vi "AccelerometerBK.vi"() -> ()   [LabVIEW 2016]
uses:
  AccelerometerSample.ctl
  Telemetry/TelemetryDataTypes.ctl
  Telemetry/TelemetryUpdateModes.ctl
  Telemetry/TelemetryFields.ctl
  <vilib>/rvi/eio/common/nirviEmuTemplateMethod_errors.vi
  <vilib>/rvi/Emulation/niFpgaGetClockAttributes.vi
  <vilib>/rvi/Emulation/niFpgaSctlEmulationGetInTimedLoop.vi
  <vilib>/rvi/Emulation/niFpgaEmulationReportErrorSimple.vi
  <vilib>/rvi/Emulation/niFpgaEmulationIsFPGAContextNoSignature.vi
  <vilib>/rvi/errors/niFpgaSetErrorForExecOnDevCompSimple.vi
  <vilib>/rvi/eio/common/nirviEmuReportErrorAndStop.vi
  <vilib>/rvi/DataTransferAndStorage/Container/Common/niFpgaContainerGetUniqueNameForEmu.vi
  <vilib>/rvi/FIFO/Fifo_Resource/nirvififoEmulationSetSize.vi
  <vilib>/rvi/FIFO/Fifo_Resource/nirviFifoEmulationQueueMgr.vi
  <instcachedir>/0/nirviFifoEmulationQueueMgr_E5CAEC123FF24DC58D834DCA3CDAA9B5.lvgen/nirviFifoEmulationQueueMgr_E5CAEC123FF24DC58D834DCA3CDAA9B5_004.vi
  <vilib>/Utility/error.llb/Clear Errors.vi
  <vilib>/rvi/FIFO/Fifo_Resource/nirvififoEmulationCreateLock.vi
  <vilib>/rvi/Emulation/niFpgaProcessEmulError.vi
  <vilib>/rvi/FIFO/Fifo_Resource/nirvififoEmulationObtainLock.vi
  <vilib>/rvi/FIFO/Fifo_Resource/nirvififoEmulationReleaseLock.vi
  <vilib>/rvi/occurrence/nirviWaitOnOccurrenceBase.vi
  <vilib>/rvi/errors/nirviReportUnexpectedCaseInternalError.vi
  <vilib>/rvi/errors/nirviReportUnexpectedCaseInternalError (U32).vi
  <instcachedir>/0/nirviFifoEmulationQueueMgr_E5CAEC123FF24DC58D834DCA3CDAA9B5.lvgen/nirviFifoEmulationQueueMgr_E5CAEC123FF24DC58D834DCA3CDAA9B5_026.vi
  <vilib>/rvi/FIFO/Fifo_Resource/nirvififoEmulationDetermineInputValidOut.vi
  <vilib>/rvi/Emulation/niFpgaCriticalErrorInLSC.vi
  <userlib>/_NI FLP Library/FPGA/outsideSCTL/FlpLib Multiply Shared Instance 0.vi
  <userlib>/_NI FLP Library/FPGA/outsideSCTL/FlpLib Add Shared Instance 0.vi
  <userlib>/_NI FLP Library/FPGA/outsideSCTL/FlpLib Subtract Shared Instance 0.vi
  <userlib>/_NI FLP Library/FPGA/outsideSCTL/FlpLib Divide Shared Instance 0.vi
  <instcachedir>/0/nirviFifoEmulationQueueMgr_E5CAEC123FF24DC58D834DCA3CDAA9B5.lvgen/nirviFifoEmulationQueueMgr_E5CAEC123FF24DC58D834DCA3CDAA9B5_024.vi
  <instcachedir>/0/nirviFifoEmulationQueueMgr_E5CAEC123FF24DC58D834DCA3CDAA9B5.lvgen/nirviFifoEmulationQueueMgr_E5CAEC123FF24DC58D834DCA3CDAA9B5_025.vi
  <vilib>/eio/EIONode/EIONode.xnode
  <vilib>/rvi/DataTransferAndStorage/Container/XNode/niFpgaContainer.xnode
  <vilib>/rvi/FIFO/Fifo_Resource/nirvififoEmulationRead.vi
  <vilib>/rvi/FIFO/Fifo_Resource/nirvififoEmulationWrite.vi
panel:
  out "Memory":T1
  out "Data":T1
  out "Sample":T2
  out "Acceleration":T1
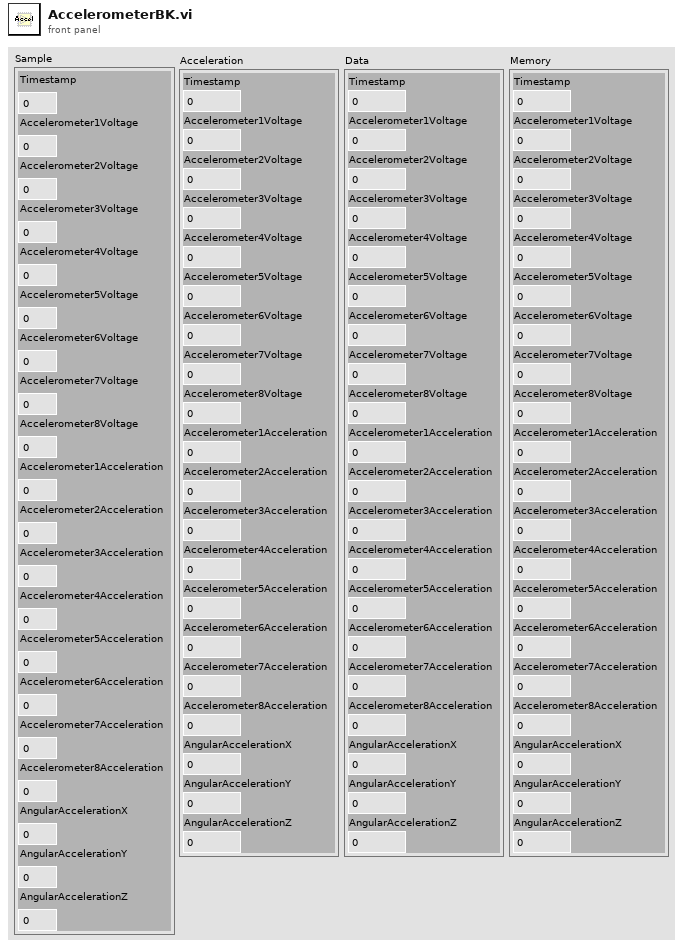
[diagram p1: front panel]
types:
  T1 = cluster{"Timestamp":u64, "Accelerometer1Voltage":sgl, "Accelerometer2Voltage":sgl, "Accelerometer3Voltage":sgl, "Accelerometer4Voltage":sgl, "Accelerometer5Voltage":sgl, "Accelerometer6Voltage":sgl, "Accelerometer7Voltage":sgl, "Accelerometer8Voltage":sgl, "Accelerometer1Acceleration":sgl, "Accelerometer2Acceleration":sgl, "Accelerometer3Acceleration":sgl, "Accelerometer4Acceleration":sgl, "Accelerometer5Acceleration":sgl, "Accelerometer6Acceleration":sgl, "Accelerometer7Acceleration":sgl, "Accelerometer8Acceleration":sgl, "AngularAccelerationX":sgl, "AngularAccelerationY":sgl, "AngularAccelerationZ":sgl}
  T2 = typedef "AccelerometerSample.ctl" = cluster{"Timestamp":u64, "Accelerometer1Voltage":sgl, "Accelerometer2Voltage":sgl, "Accelerometer3Voltage":sgl, "Accelerometer4Voltage":sgl, "Accelerometer5Voltage":sgl, "Accelerometer6Voltage":sgl, "Accelerometer7Voltage":sgl, "Accelerometer8Voltage":sgl, "Accelerometer1Acceleration":sgl, "Accelerometer2Acceleration":sgl, "Accelerometer3Acceleration":sgl, "Accelerometer4Acceleration":sgl, "Accelerometer5Acceleration":sgl, "Accelerometer6Acceleration":sgl, "Accelerometer7Acceleration":sgl, "Accelerometer8Acceleration":sgl, "AngularAccelerationX":sgl, "AngularAccelerationY":sgl, "AngularAccelerationZ":sgl}
  T3 = typedef "TelemetryFields.ctl" = enum16{"InclinometerErrorCode", "InclinometerTxBytes", "InclinometerRxBytes", "InclinometerTxFrames", "InclinometerRxFrames", "InclinometerTimestamp", "InclinometerAngle", "DisplacementErrorCode", "DisplacementTxBytes", "DisplacementRxBytes", "DisplacementTxFrames", "DisplacementRxFrames", "DisplacementTimestamp", "Displacement1", "Displacement2", "Displacement3", "Displacement4", "Displacement5", "Displacement6", "Displacement7", "Displacement8", "AccelerometerSampleCount", "AccelerometerTimestamp", "AccelerometerRaw1", "AccelerometerRaw2", "AccelerometerRaw3", "AccelerometerRaw4", "AccelerometerRaw5", "AccelerometerRaw6", "AccelerometerRaw7", "AccelerometerRaw8", "AccelerometerEng1", "AccelerometerEng2", "AccelerometerEng3", "AccelerometerEng4", "AccelerometerEng5", "AccelerometerEng6", "AccelerometerEng7", "AccelerometerEng8", "AngularAccelerationX", "AngularAccelerationY", "AngularAccelerationZ"}
  T4 = typedef "TelemetryUpdateModes.ctl" = enum8{"=", "+", "-", "|"}
  T5 = typedef "TelemetryDataTypes.ctl" = enum8{"U8", "U16", "U32", "U64", "I8", "I16", "I32", "I64", "SGL"}
  T6 = typedef "TelemetryUpdateData.ctl" = cluster{"DataType":T5, "Mode":T4, "Field":T3, "Data":u64}
  T7 = typedef "TelemetryUpdateDataSGL.ctl" = cluster{"Mode":T4, "Field":T3, "Data":sgl}
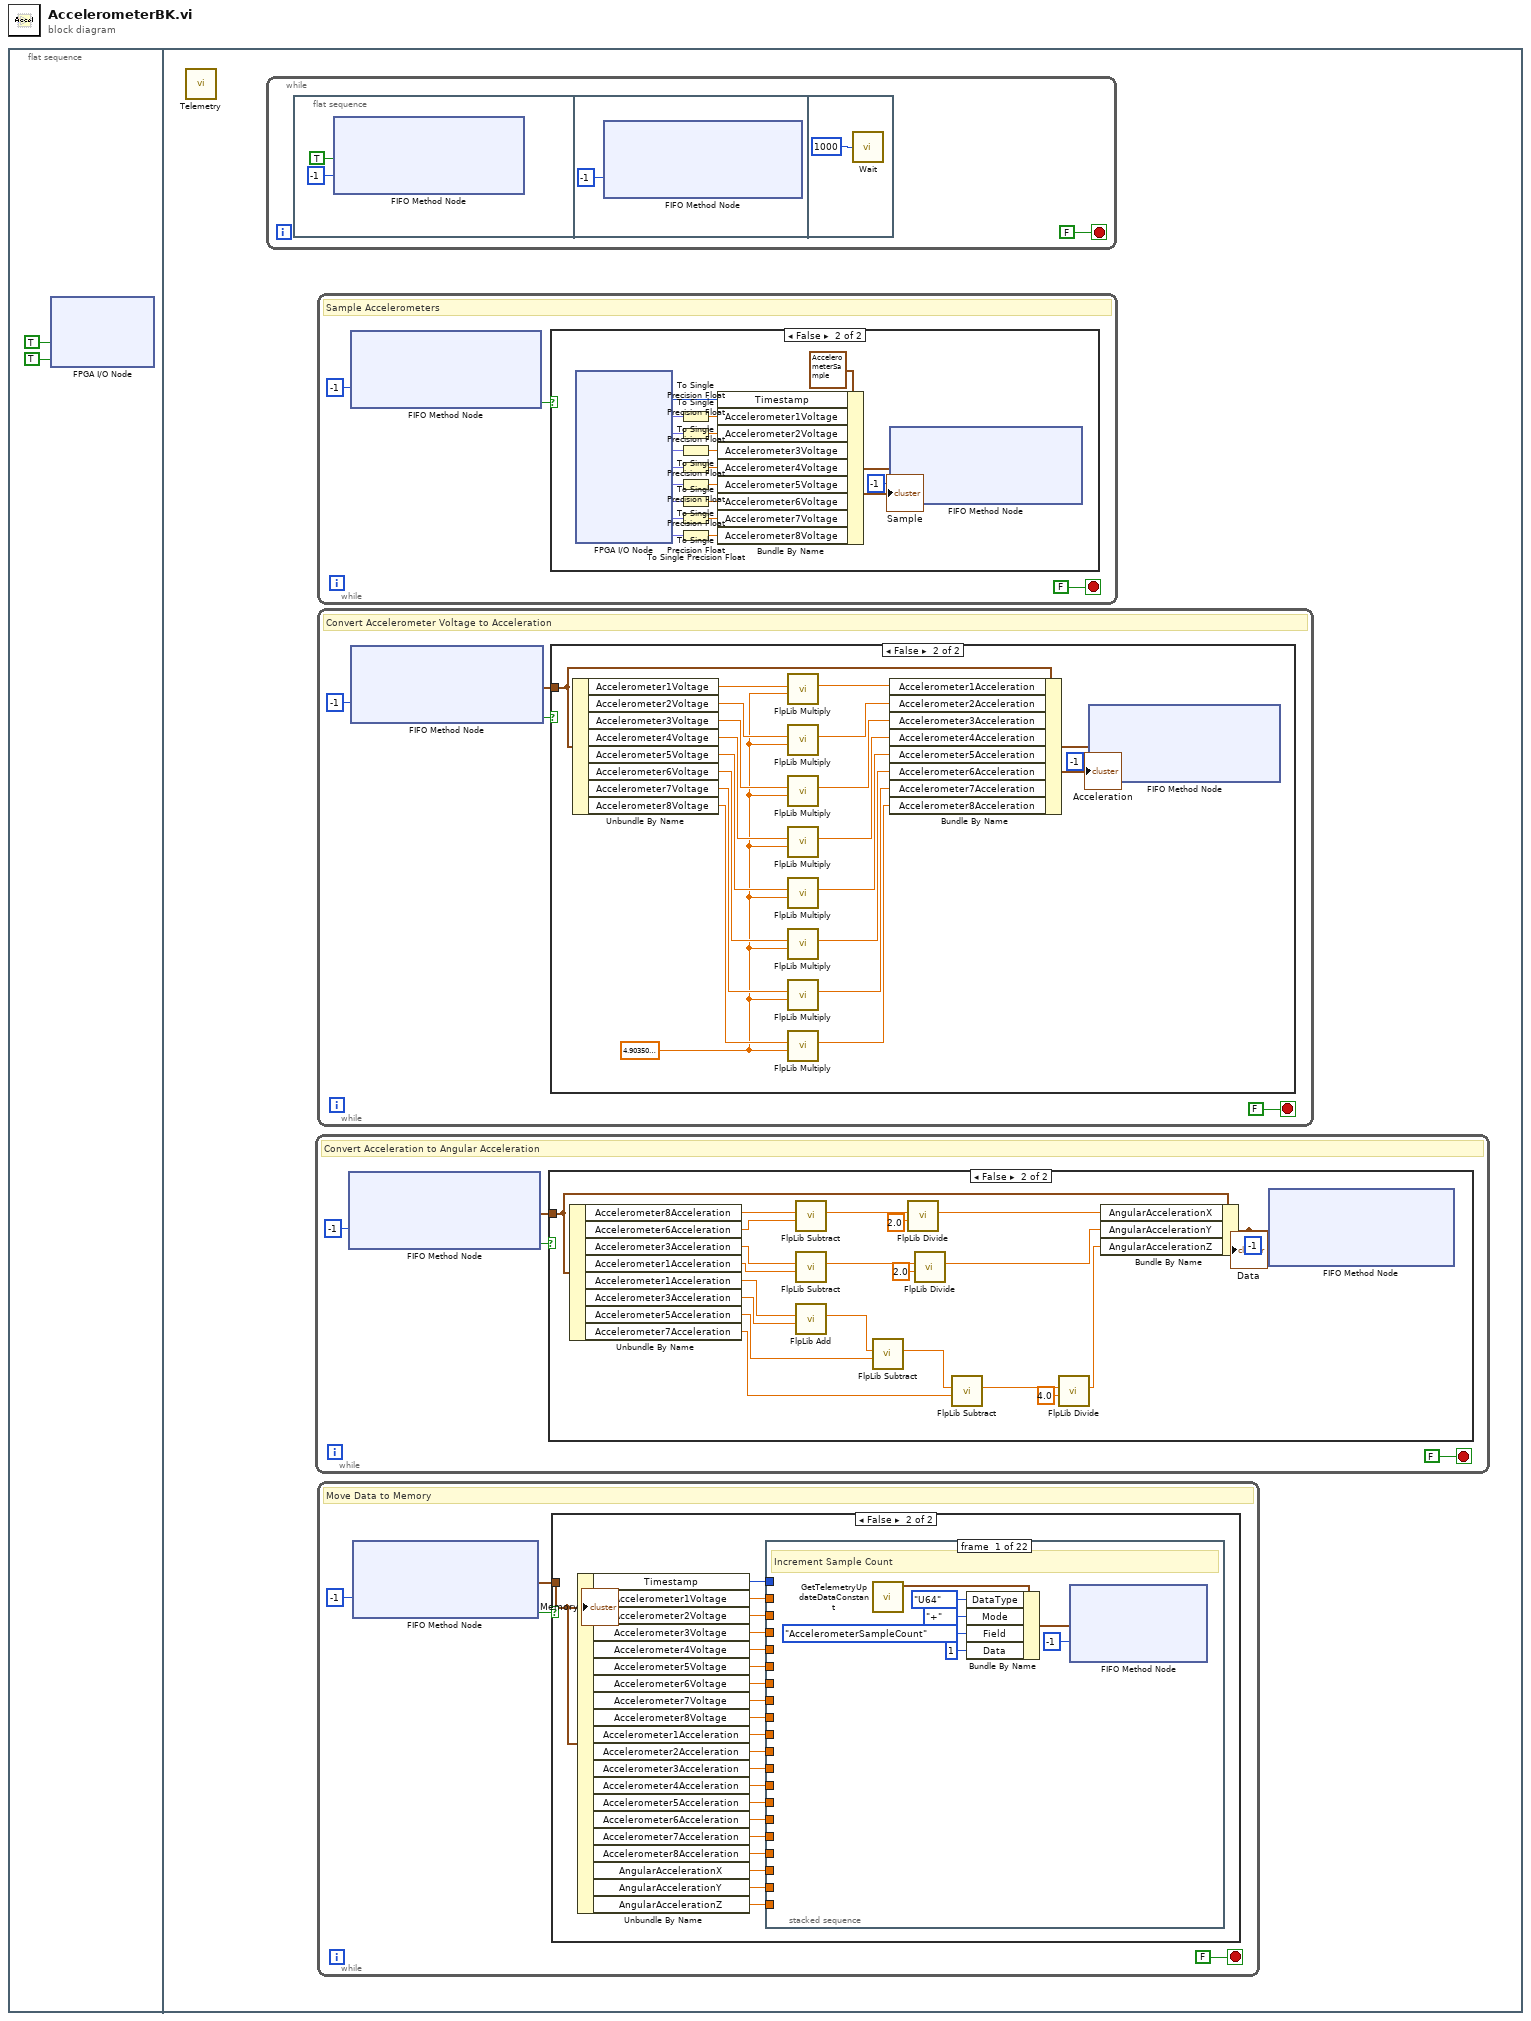
[diagram p0: block diagram]
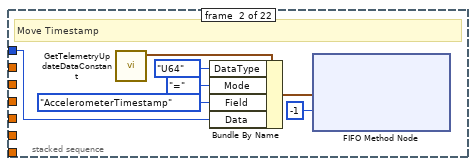
[diagram p3: hidden frame]
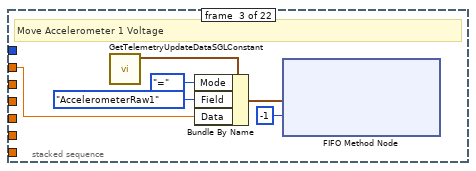
[diagram p4: hidden frame]
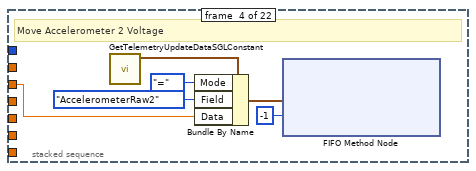
[diagram p5: hidden frame]
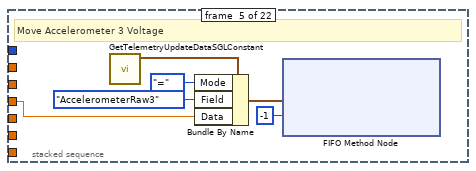
[diagram p6: hidden frame]
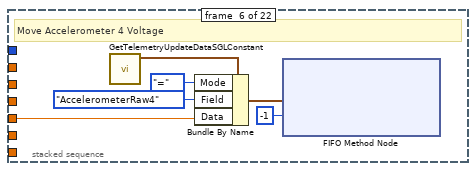
[diagram p7: hidden frame]
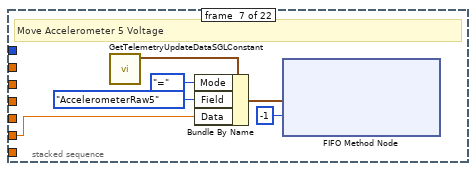
[diagram p8: hidden frame]
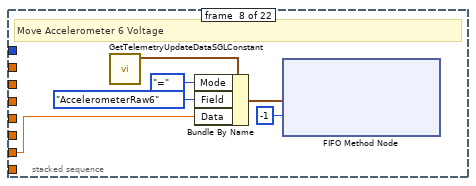
[diagram p9: hidden frame]
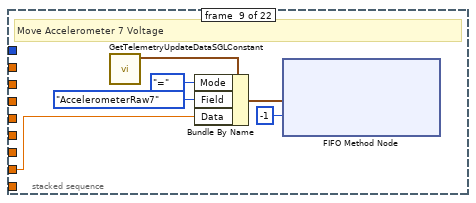
[diagram p10: hidden frame]
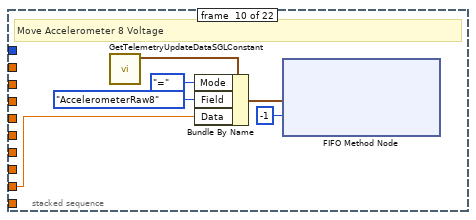
[diagram p11: hidden frame]
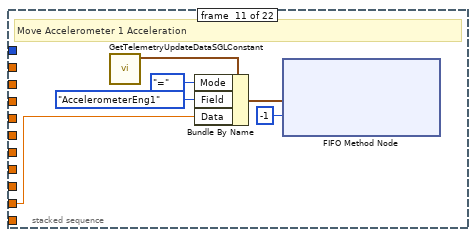
[diagram p12: hidden frame]
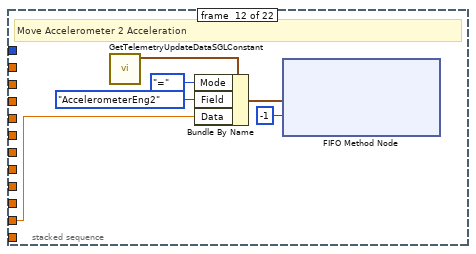
[diagram p13: hidden frame]
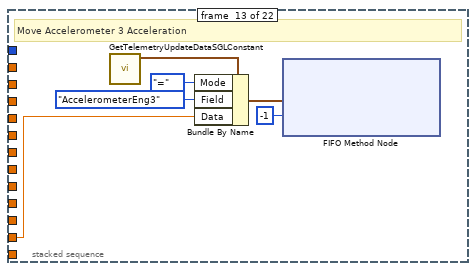
[diagram p14: hidden frame]
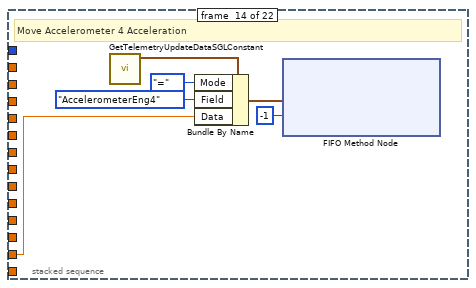
[diagram p15: hidden frame]
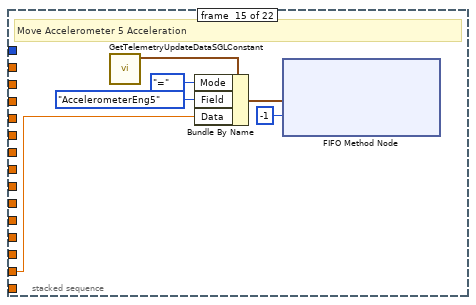
[diagram p16: hidden frame]
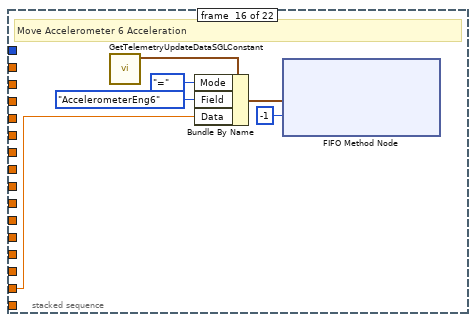
[diagram p17: hidden frame]
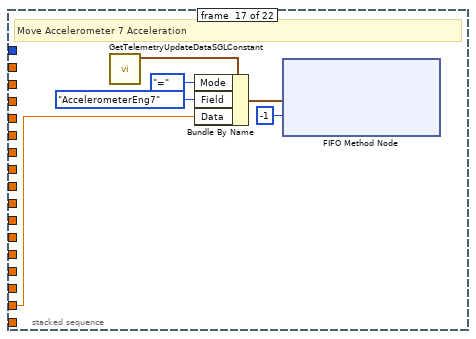
[diagram p18: hidden frame]
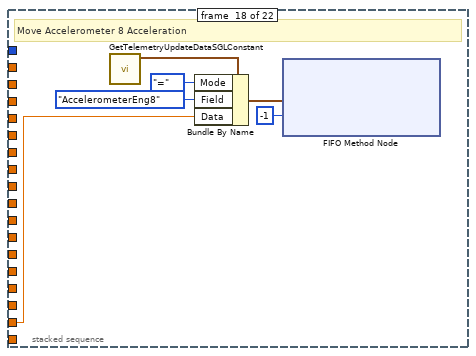
[diagram p19: hidden frame]
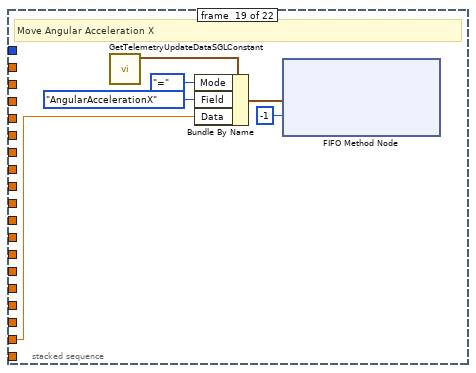
[diagram p20: hidden frame]
diagram:
  n1 = flat-sequence {
    frame #0 {
      n2 = xnode "FPGA I/O Node"("Mod1/Start"=TRUE, "Mod2/Start"=TRUE) -> ()  [unwired: 3 in, 4 out]
    }
    frame #1 {
      n3 = call "Telemetry.vi"() -> ()  [unwired: 12 in]
      n4 = while {
        stop <- FALSE stop-if-true
        n5 = flat-sequence {
          frame #0 {
            n6 = xnode ("FIFO Method Node")("Element"=TRUE, "Timeout"=-1) -> ()  [unwired: 1 in, 2 out]
          }
          frame #1 {
            n7 = xnode ("FIFO Method Node")("Timeout"=-1) -> ()  [unwired: 1 in, 3 out]
          }
          frame #2 {
            n8 = call "Wait"("Count(uSec)"=u32 1000 ("Count(mSec)")) -> ()  [unwired: 1 out]
          }
        }
      }
      n9 = while {
        stop <- FALSE stop-if-true
        # "Convert Acceleration to Angular Acceleration"
        n10 = xnode ("FIFO Method Node")("Timeout"=-1) -> ("Element"=w164:T1, "Timed Out?"=w165:bool)  [unwired: 1 in, 1 out]
        n11 = case shown="False" w165 {
          tunnel: w164 -> [_ w180]
          frame True {
          }
          frame False {
            n12 = Unbundle By Name(w180) -> ("Accelerometer8Acceleration"=w179:sgl, "Accelerometer6Acceleration"=w178:sgl, "Accelerometer3Acceleration"=w176:sgl, "Accelerometer1Acceleration"=w175:sgl, "Accelerometer1Acceleration"=w174:sgl, "Accelerometer3Acceleration"=w173:sgl, "Accelerometer5Acceleration"=w172:sgl, "Accelerometer7Acceleration"=w171:sgl)
            n13 = call-poly <userlib>:"FlpLib Subtract.vi"("y"=w178, "x"=w179) -> ("x-y"=w188:sgl)  [unwired: 5 in]
            n14 = call-poly <userlib>:"FlpLib Subtract.vi"("y"=w175, "x"=w176) -> ("x-y"=w185:sgl)  [unwired: 5 in]
            n15 = call-poly <userlib>:"FlpLib Add.vi"("y"=w173, "x"=w174) -> ("x+y"=w184:sgl)  [unwired: 5 in]
            n16 = call-poly <userlib>:"FlpLib Subtract.vi"("y"=w172, "x"=w184) -> ("x-y"=w183:sgl)  [unwired: 5 in]
            n17 = call-poly <userlib>:"FlpLib Divide.vi"("y"=sgl 2.0, "x"=w188) -> ("x/y"=w177:sgl)  [unwired: 5 in]
            n18 = call-poly <userlib>:"FlpLib Divide.vi"("y"=sgl 2.0, "x"=w185) -> ("x/y"=w170:sgl)  [unwired: 5 in]
            n19 = call-poly <userlib>:"FlpLib Subtract.vi"("y"=w171, "x"=w183) -> ("x-y"=w181:sgl)  [unwired: 5 in]
            n20 = call-poly <userlib>:"FlpLib Divide.vi"("y"=sgl 4.0, "x"=w181) -> ("x/y"=w169:sgl)  [unwired: 5 in]
            n21 = Bundle By Name(cluster=w180, "AngularAccelerationX"=w177, "AngularAccelerationY"=w170, "AngularAccelerationZ"=w169) -> (w167:T1)
            "Data" <- w167
            n22 = xnode ("FIFO Method Node")("Element"=w167, "Timeout"=-1) -> ()  [unwired: 1 in, 2 out]
          }
        }
      }
      n23 = while {
        stop <- FALSE stop-if-true
        # "Sample Accelerometers"
        n24 = xnode ("FIFO Method Node")("Timeout"=-1) -> ("Timed Out?"=w214:bool)  [unwired: 1 in, 2 out]
        n25 = case shown="False" w214 {
          frame True {
          }
          frame False {
            n26 = xnode "FPGA I/O Node"() -> ("Time"=w227:u64, "Mod1/AI0"=w235:fxp<+/-,24,5>, "Mod1/AI1"=w234:fxp<+/-,24,5>, "Mod1/AI2"=w233:fxp<+/-,24,5>, "Mod1/AI3"=w232:fxp<+/-,24,5>, "Mod2/AI0"=w231:fxp<+/-,24,5>, "Mod2/AI1"=w230:fxp<+/-,24,5>, "Mod2/AI2"=w229:fxp<+/-,24,5>, "Mod2/AI3"=w228:fxp<+/-,24,5>)  [unwired: 9 in, 9 out]
            n27 = To Single Precision Float(number=w235) -> (single precision float=w226:sgl)
            n28 = To Single Precision Float(number=w234) -> (single precision float=w225:sgl)
            n29 = To Single Precision Float(number=w233) -> (single precision float=w224:sgl)
            n30 = To Single Precision Float(number=w232) -> (single precision float=w223:sgl)
            n31 = To Single Precision Float(number=w231) -> (single precision float=w222:sgl)
            n32 = To Single Precision Float(number=w230) -> (single precision float=w221:sgl)
            n33 = To Single Precision Float(number=w229) -> (single precision float=w220:sgl)
            n34 = To Single Precision Float(number=w228) -> (single precision float=w219:sgl)
            n35 = Bundle By Name(cluster=T2 {"Timestamp"=0, "Accelerometer1Voltage"=0.0, "Accelerometer2Voltage"=0.0, "Accelerometer3Voltage"=0.0, "Accelerometer4Voltage"=0.0, "Accelerometer5Voltage"=0.0, "Accelerometer6Voltage"=0.0, "Accelerometer7Voltage"=0.0, "Accelerometer8Voltage"=0.0, "Accelerometer1Acceleration"=0.0, "Accelerometer2Acceleration"=0.0, "Accelerometer3Acceleration"=0.0, "Accelerometer4Acceleration"=0.0, "Accelerometer5Acceleration"=0.0, "Accelerometer6Acceleration"=0.0, "Accelerometer7Acceleration"=0.0, "Accelerometer8Acceleration"=0.0, "AngularAccelerationX"=0.0, "AngularAccelerationY"=0.0, "AngularAccelerationZ"=0.0} ("AccelerometerSample"), "Timestamp"=w227, "Accelerometer1Voltage"=w226, "Accelerometer2Voltage"=w225, "Accelerometer3Voltage"=w224, "Accelerometer4Voltage"=w223, "Accelerometer5Voltage"=w222, "Accelerometer6Voltage"=w221, "Accelerometer7Voltage"=w220, "Accelerometer8Voltage"=w219) -> (w218:T2)
            "Sample" <- w218
            n36 = xnode ("FIFO Method Node")("Element"=w218, "Timeout"=-1) -> ()  [unwired: 1 in, 2 out]
          }
        }
      }
      n37 = while {
        stop <- FALSE stop-if-true
        # "Convert Accelerometer Voltage to Acceleration"
        n38 = xnode ("FIFO Method Node")("Timeout"=-1) -> ("Element"=w189:T1, "Timed Out?"=w191:bool)  [unwired: 1 in, 1 out]
        n39 = case shown="False" w191 {
          tunnel: w189 -> [_ w202]
          frame True {
          }
          frame False {
            w203 = sgl 4.9035 ("y")
            n40 = Unbundle By Name(w202) -> ("Accelerometer1Voltage"=w211:sgl, "Accelerometer2Voltage"=w204:sgl, "Accelerometer3Voltage"=w205:sgl, "Accelerometer4Voltage"=w206:sgl, "Accelerometer5Voltage"=w207:sgl, "Accelerometer6Voltage"=w208:sgl, "Accelerometer7Voltage"=w209:sgl, "Accelerometer8Voltage"=w210:sgl)
            n41 = call-poly <userlib>:"FlpLib Multiply.vi"("y"=w203, "x"=w211) -> ("x*y"=w200:sgl)  [unwired: 5 in]
            n42 = call-poly <userlib>:"FlpLib Multiply.vi"("y"=w203, "x"=w204) -> ("x*y"=w193:sgl)  [unwired: 5 in]
            n43 = call-poly <userlib>:"FlpLib Multiply.vi"("y"=w203, "x"=w205) -> ("x*y"=w194:sgl)  [unwired: 5 in]
            n44 = call-poly <userlib>:"FlpLib Multiply.vi"("y"=w203, "x"=w206) -> ("x*y"=w195:sgl)  [unwired: 5 in]
            n45 = call-poly <userlib>:"FlpLib Multiply.vi"("y"=w203, "x"=w207) -> ("x*y"=w196:sgl)  [unwired: 5 in]
            n46 = call-poly <userlib>:"FlpLib Multiply.vi"("y"=w203, "x"=w208) -> ("x*y"=w197:sgl)  [unwired: 5 in]
            n47 = call-poly <userlib>:"FlpLib Multiply.vi"("y"=w203, "x"=w209) -> ("x*y"=w198:sgl)  [unwired: 5 in]
            n48 = call-poly <userlib>:"FlpLib Multiply.vi"("y"=w203, "x"=w210) -> ("x*y"=w199:sgl)  [unwired: 5 in]
            n49 = Bundle By Name(cluster=w202, "Accelerometer1Acceleration"=w200, "Accelerometer2Acceleration"=w193, "Accelerometer3Acceleration"=w194, "Accelerometer4Acceleration"=w195, "Accelerometer5Acceleration"=w196, "Accelerometer6Acceleration"=w197, "Accelerometer7Acceleration"=w198, "Accelerometer8Acceleration"=w199) -> (w201:T1)
            "Acceleration" <- w201
            n50 = xnode ("FIFO Method Node")("Element"=w201, "Timeout"=-1) -> ()  [unwired: 1 in, 2 out]
          }
        }
      }
      n51 = while {
        stop <- FALSE stop-if-true
        # "Move Data to Memory"
        n52 = xnode ("FIFO Method Node")("Timeout"=-1) -> ("Element"=w9:T1, "Timed Out?"=w10:bool)  [unwired: 1 in, 1 out]
        n53 = case shown="False" w10 {
          tunnel: w9 -> [_ w32]
          frame True {
          }
          frame False {
            n54 = Unbundle By Name(w32) -> ("Timestamp"=w31:u64, "Accelerometer1Voltage"=w30:sgl, "Accelerometer2Voltage"=w29:sgl, "Accelerometer3Voltage"=w28:sgl, "Accelerometer4Voltage"=w27:sgl, "Accelerometer5Voltage"=w26:sgl, "Accelerometer6Voltage"=w25:sgl, "Accelerometer7Voltage"=w24:sgl, "Accelerometer8Voltage"=w23:sgl, "Accelerometer1Acceleration"=w22:sgl, "Accelerometer2Acceleration"=w21:sgl, "Accelerometer3Acceleration"=w20:sgl, "Accelerometer4Acceleration"=w19:sgl, "Accelerometer5Acceleration"=w18:sgl, "Accelerometer6Acceleration"=w17:sgl, "Accelerometer7Acceleration"=w16:sgl, "Accelerometer8Acceleration"=w15:sgl, "AngularAccelerationX"=w14:sgl, "AngularAccelerationY"=w13:sgl, "AngularAccelerationZ"=w12:sgl)
            n55 = stacked-sequence {
              tunnel: w31 -> [_ w40 _ _ _ _ _ _ _ _ _ _ _ _ _ _ _ _ _ _ _ _]
              tunnel: w30 -> [_ _ w47 _ _ _ _ _ _ _ _ _ _ _ _ _ _ _ _ _ _ _]
              tunnel: w29 -> [_ _ _ w53 _ _ _ _ _ _ _ _ _ _ _ _ _ _ _ _ _ _]
              tunnel: w28 -> [_ _ _ _ w59 _ _ _ _ _ _ _ _ _ _ _ _ _ _ _ _ _]
              tunnel: w27 -> [_ _ _ _ _ w65 _ _ _ _ _ _ _ _ _ _ _ _ _ _ _ _]
              tunnel: w26 -> [_ _ _ _ _ _ w71 _ _ _ _ _ _ _ _ _ _ _ _ _ _ _]
              tunnel: w25 -> [_ _ _ _ _ _ _ w77 _ _ _ _ _ _ _ _ _ _ _ _ _ _]
              tunnel: w24 -> [_ _ _ _ _ _ _ _ w83 _ _ _ _ _ _ _ _ _ _ _ _ _]
              tunnel: w23 -> [_ _ _ _ _ _ _ _ _ w89 _ _ _ _ _ _ _ _ _ _ _ _]
              tunnel: w22 -> [_ _ _ _ _ _ _ _ _ _ w95 _ _ _ _ _ _ _ _ _ _ _]
              tunnel: w21 -> [_ _ _ _ _ _ _ _ _ _ _ w101 _ _ _ _ _ _ _ _ _ _]
              tunnel: w20 -> [_ _ _ _ _ _ _ _ _ _ _ _ w107 _ _ _ _ _ _ _ _ _]
              tunnel: w19 -> [_ _ _ _ _ _ _ _ _ _ _ _ _ w113 _ _ _ _ _ _ _ _]
              tunnel: w18 -> [_ _ _ _ _ _ _ _ _ _ _ _ _ _ w119 _ _ _ _ _ _ _]
              tunnel: w17 -> [_ _ _ _ _ _ _ _ _ _ _ _ _ _ _ w125 _ _ _ _ _ _]
              tunnel: w16 -> [_ _ _ _ _ _ _ _ _ _ _ _ _ _ _ _ w131 _ _ _ _ _]
              tunnel: w15 -> [_ _ _ _ _ _ _ _ _ _ _ _ _ _ _ _ _ w137 _ _ _ _]
              tunnel: w14 -> [_ _ _ _ _ _ _ _ _ _ _ _ _ _ _ _ _ _ w143 _ _ _]
              tunnel: w13 -> [_ _ _ _ _ _ _ _ _ _ _ _ _ _ _ _ _ _ _ w149 _ _]
              tunnel: w12 -> [_ _ _ _ _ _ _ _ _ _ _ _ _ _ _ _ _ _ _ _ w155 _]
              frame #0 {
                # "Increment Sample Count"
                n56 = call "GetTelemetryUpdateDataConstant.vi"() -> ("TelemetryUpdateData"=w34:T6)  [unwired: 11 in]
                n57 = Bundle By Name(cluster=w34, "DataType"=TelemetryDataTypes."U64" ("TelemetryDataTypes"), "Mode"=TelemetryUpdateModes."+" ("TelemetryUpdateModes"), "Field"=TelemetryFields."AccelerometerSampleCount" ("TelemetryFields"), "Data"=u64 1) -> (w36:T6)
                n58 = xnode ("FIFO Method Node")("Element"=w36, "Timeout"=-1) -> ()  [unwired: 1 in, 2 out]
              }
              frame #1 {
                # "Move Timestamp"
                n59 = call "GetTelemetryUpdateDataConstant.vi"() -> ("TelemetryUpdateData"=w41:T6)  [unwired: 11 in]
                n60 = Bundle By Name(cluster=w41, "DataType"=TelemetryDataTypes."U64" ("TelemetryDataTypes"), "Mode"=TelemetryUpdateModes."=" ("TelemetryUpdateModes"), "Field"=TelemetryFields."AccelerometerTimestamp" ("TelemetryFields"), "Data"=w40) -> (w43:T6)
                n61 = xnode ("FIFO Method Node")("Element"=w43, "Timeout"=-1) -> ()  [unwired: 1 in, 2 out]
              }
              frame #2 {
                # "Move Accelerometer 1 Voltage"
                n62 = call "GetTelemetryUpdateDataSGLConstant.vi"() -> ("TelemetryUpdateDataSGL"=w51:T7)  [unwired: 11 in]
                n63 = Bundle By Name(cluster=w51, "Mode"=TelemetryUpdateModes."=" ("TelemetryUpdateModes"), "Field"=TelemetryFields."AccelerometerRaw1" ("TelemetryFields"), "Data"=w47) -> (w52:T7)
                n64 = xnode ("FIFO Method Node")("Element"=w52, "Timeout"=-1) -> ()  [unwired: 1 in, 2 out]
              }
              frame #3 {
                # "Move Accelerometer 2 Voltage"
                n65 = call "GetTelemetryUpdateDataSGLConstant.vi"() -> ("TelemetryUpdateDataSGL"=w57:T7)  [unwired: 11 in]
                n66 = Bundle By Name(cluster=w57, "Mode"=TelemetryUpdateModes."=" ("TelemetryUpdateModes"), "Field"=TelemetryFields."AccelerometerRaw2" ("TelemetryFields"), "Data"=w53) -> (w58:T7)
                n67 = xnode ("FIFO Method Node")("Element"=w58, "Timeout"=-1) -> ()  [unwired: 1 in, 2 out]
              }
              frame #4 {
                # "Move Accelerometer 3 Voltage"
                n68 = call "GetTelemetryUpdateDataSGLConstant.vi"() -> ("TelemetryUpdateDataSGL"=w63:T7)  [unwired: 11 in]
                n69 = Bundle By Name(cluster=w63, "Mode"=TelemetryUpdateModes."=" ("TelemetryUpdateModes"), "Field"=TelemetryFields."AccelerometerRaw3" ("TelemetryFields"), "Data"=w59) -> (w64:T7)
                n70 = xnode ("FIFO Method Node")("Element"=w64, "Timeout"=-1) -> ()  [unwired: 1 in, 2 out]
              }
              frame #5 {
                # "Move Accelerometer 4 Voltage"
                n71 = call "GetTelemetryUpdateDataSGLConstant.vi"() -> ("TelemetryUpdateDataSGL"=w69:T7)  [unwired: 11 in]
                n72 = Bundle By Name(cluster=w69, "Mode"=TelemetryUpdateModes."=" ("TelemetryUpdateModes"), "Field"=TelemetryFields."AccelerometerRaw4" ("TelemetryFields"), "Data"=w65) -> (w70:T7)
                n73 = xnode ("FIFO Method Node")("Element"=w70, "Timeout"=-1) -> ()  [unwired: 1 in, 2 out]
              }
              frame #6 {
                # "Move Accelerometer 5 Voltage"
                n74 = call "GetTelemetryUpdateDataSGLConstant.vi"() -> ("TelemetryUpdateDataSGL"=w75:T7)  [unwired: 11 in]
                n75 = Bundle By Name(cluster=w75, "Mode"=TelemetryUpdateModes."=" ("TelemetryUpdateModes"), "Field"=TelemetryFields."AccelerometerRaw5" ("TelemetryFields"), "Data"=w71) -> (w76:T7)
                n76 = xnode ("FIFO Method Node")("Element"=w76, "Timeout"=-1) -> ()  [unwired: 1 in, 2 out]
              }
              frame #7 {
                # "Move Accelerometer 6 Voltage"
                n77 = call "GetTelemetryUpdateDataSGLConstant.vi"() -> ("TelemetryUpdateDataSGL"=w81:T7)  [unwired: 11 in]
                n78 = Bundle By Name(cluster=w81, "Mode"=TelemetryUpdateModes."=" ("TelemetryUpdateModes"), "Field"=TelemetryFields."AccelerometerRaw6" ("TelemetryFields"), "Data"=w77) -> (w82:T7)
                n79 = xnode ("FIFO Method Node")("Element"=w82, "Timeout"=-1) -> ()  [unwired: 1 in, 2 out]
              }
              frame #8 {
                # "Move Accelerometer 7 Voltage"
                n80 = call "GetTelemetryUpdateDataSGLConstant.vi"() -> ("TelemetryUpdateDataSGL"=w87:T7)  [unwired: 11 in]
                n81 = Bundle By Name(cluster=w87, "Mode"=TelemetryUpdateModes."=" ("TelemetryUpdateModes"), "Field"=TelemetryFields."AccelerometerRaw7" ("TelemetryFields"), "Data"=w83) -> (w88:T7)
                n82 = xnode ("FIFO Method Node")("Element"=w88, "Timeout"=-1) -> ()  [unwired: 1 in, 2 out]
              }
              frame #9 {
                # "Move Accelerometer 8 Voltage"
                n83 = call "GetTelemetryUpdateDataSGLConstant.vi"() -> ("TelemetryUpdateDataSGL"=w93:T7)  [unwired: 11 in]
                n84 = Bundle By Name(cluster=w93, "Mode"=TelemetryUpdateModes."=" ("TelemetryUpdateModes"), "Field"=TelemetryFields."AccelerometerRaw8" ("TelemetryFields"), "Data"=w89) -> (w94:T7)
                n85 = xnode ("FIFO Method Node")("Element"=w94, "Timeout"=-1) -> ()  [unwired: 1 in, 2 out]
              }
              frame #10 {
                # "Move Accelerometer 1 Acceleration"
                n86 = call "GetTelemetryUpdateDataSGLConstant.vi"() -> ("TelemetryUpdateDataSGL"=w99:T7)  [unwired: 11 in]
                n87 = Bundle By Name(cluster=w99, "Mode"=TelemetryUpdateModes."=" ("TelemetryUpdateModes"), "Field"=TelemetryFields."AccelerometerEng1" ("TelemetryFields"), "Data"=w95) -> (w100:T7)
                n88 = xnode ("FIFO Method Node")("Element"=w100, "Timeout"=-1) -> ()  [unwired: 1 in, 2 out]
              }
              frame #11 {
                # "Move Accelerometer 2 Acceleration"
                n89 = call "GetTelemetryUpdateDataSGLConstant.vi"() -> ("TelemetryUpdateDataSGL"=w105:T7)  [unwired: 11 in]
                n90 = Bundle By Name(cluster=w105, "Mode"=TelemetryUpdateModes."=" ("TelemetryUpdateModes"), "Field"=TelemetryFields."AccelerometerEng2" ("TelemetryFields"), "Data"=w101) -> (w106:T7)
                n91 = xnode ("FIFO Method Node")("Element"=w106, "Timeout"=-1) -> ()  [unwired: 1 in, 2 out]
              }
              frame #12 {
                # "Move Accelerometer 3 Acceleration"
                n92 = call "GetTelemetryUpdateDataSGLConstant.vi"() -> ("TelemetryUpdateDataSGL"=w111:T7)  [unwired: 11 in]
                n93 = Bundle By Name(cluster=w111, "Mode"=TelemetryUpdateModes."=" ("TelemetryUpdateModes"), "Field"=TelemetryFields."AccelerometerEng3" ("TelemetryFields"), "Data"=w107) -> (w112:T7)
                n94 = xnode ("FIFO Method Node")("Element"=w112, "Timeout"=-1) -> ()  [unwired: 1 in, 2 out]
              }
              frame #13 {
                # "Move Accelerometer 4 Acceleration"
                n95 = call "GetTelemetryUpdateDataSGLConstant.vi"() -> ("TelemetryUpdateDataSGL"=w117:T7)  [unwired: 11 in]
                n96 = Bundle By Name(cluster=w117, "Mode"=TelemetryUpdateModes."=" ("TelemetryUpdateModes"), "Field"=TelemetryFields."AccelerometerEng4" ("TelemetryFields"), "Data"=w113) -> (w118:T7)
                n97 = xnode ("FIFO Method Node")("Element"=w118, "Timeout"=-1) -> ()  [unwired: 1 in, 2 out]
              }
              frame #14 {
                # "Move Accelerometer 5 Acceleration"
                n98 = call "GetTelemetryUpdateDataSGLConstant.vi"() -> ("TelemetryUpdateDataSGL"=w123:T7)  [unwired: 11 in]
                n99 = Bundle By Name(cluster=w123, "Mode"=TelemetryUpdateModes."=" ("TelemetryUpdateModes"), "Field"=TelemetryFields."AccelerometerEng5" ("TelemetryFields"), "Data"=w119) -> (w124:T7)
                n100 = xnode ("FIFO Method Node")("Element"=w124, "Timeout"=-1) -> ()  [unwired: 1 in, 2 out]
              }
              frame #15 {
                # "Move Accelerometer 6 Acceleration"
                n101 = call "GetTelemetryUpdateDataSGLConstant.vi"() -> ("TelemetryUpdateDataSGL"=w129:T7)  [unwired: 11 in]
                n102 = Bundle By Name(cluster=w129, "Mode"=TelemetryUpdateModes."=" ("TelemetryUpdateModes"), "Field"=TelemetryFields."AccelerometerEng6" ("TelemetryFields"), "Data"=w125) -> (w130:T7)
                n103 = xnode ("FIFO Method Node")("Element"=w130, "Timeout"=-1) -> ()  [unwired: 1 in, 2 out]
              }
              frame #16 {
                # "Move Accelerometer 7 Acceleration"
                n104 = call "GetTelemetryUpdateDataSGLConstant.vi"() -> ("TelemetryUpdateDataSGL"=w135:T7)  [unwired: 11 in]
                n105 = Bundle By Name(cluster=w135, "Mode"=TelemetryUpdateModes."=" ("TelemetryUpdateModes"), "Field"=TelemetryFields."AccelerometerEng7" ("TelemetryFields"), "Data"=w131) -> (w136:T7)
                n106 = xnode ("FIFO Method Node")("Element"=w136, "Timeout"=-1) -> ()  [unwired: 1 in, 2 out]
              }
              frame #17 {
                # "Move Accelerometer 8 Acceleration"
                n107 = call "GetTelemetryUpdateDataSGLConstant.vi"() -> ("TelemetryUpdateDataSGL"=w141:T7)  [unwired: 11 in]
                n108 = Bundle By Name(cluster=w141, "Mode"=TelemetryUpdateModes."=" ("TelemetryUpdateModes"), "Field"=TelemetryFields."AccelerometerEng8" ("TelemetryFields"), "Data"=w137) -> (w142:T7)
                n109 = xnode ("FIFO Method Node")("Element"=w142, "Timeout"=-1) -> ()  [unwired: 1 in, 2 out]
              }
              frame #18 {
                # "Move Angular Acceleration X"
                n110 = call "GetTelemetryUpdateDataSGLConstant.vi"() -> ("TelemetryUpdateDataSGL"=w147:T7)  [unwired: 11 in]
                n111 = Bundle By Name(cluster=w147, "Mode"=TelemetryUpdateModes."=" ("TelemetryUpdateModes"), "Field"=TelemetryFields."AngularAccelerationX" ("TelemetryFields"), "Data"=w143) -> (w148:T7)
                n112 = xnode ("FIFO Method Node")("Element"=w148, "Timeout"=-1) -> ()  [unwired: 1 in, 2 out]
              }
              frame #19 {
                # "Move Angular Acceleration Y"
                n113 = call "GetTelemetryUpdateDataSGLConstant.vi"() -> ("TelemetryUpdateDataSGL"=w153:T7)  [unwired: 11 in]
                n114 = Bundle By Name(cluster=w153, "Mode"=TelemetryUpdateModes."=" ("TelemetryUpdateModes"), "Field"=TelemetryFields."AngularAccelerationY" ("TelemetryFields"), "Data"=w149) -> (w154:T7)
                n115 = xnode ("FIFO Method Node")("Element"=w154, "Timeout"=-1) -> ()  [unwired: 1 in, 2 out]
              }
              frame #20 {
                # "Move Angular Acceleration Z"
                n116 = call "GetTelemetryUpdateDataSGLConstant.vi"() -> ("TelemetryUpdateDataSGL"=w159:T7)  [unwired: 11 in]
                n117 = Bundle By Name(cluster=w159, "Mode"=TelemetryUpdateModes."=" ("TelemetryUpdateModes"), "Field"=TelemetryFields."AngularAccelerationZ" ("TelemetryFields"), "Data"=w155) -> (w160:T7)
                n118 = xnode ("FIFO Method Node")("Element"=w160, "Timeout"=-1) -> ()  [unwired: 1 in, 2 out]
              }
              frame #21 {
                # "Notify Processing Complete"
                n119 = xnode ("FIFO Method Node")("Element"=TRUE, "Timeout"=-1) -> ()  [unwired: 1 in, 2 out]
              }
            }
            "Memory" <- w32
          }
        }
      }
    }
  }
